vi "Add Attribute To Tree.vi"(6 "Display Name":string="Root::AcquisitionControl::AcquisitionStart", 8 "Error In":errorcluster, 9 "Active Item:Symbol Index":i32, 10 "Attribute Name":string="Root::AcquisitionControl::AcquisitionStart", 11 "Attribute Table In":refnum<vi>) -> (0 "Error Out":errorcluster, 3 "Attribute Table Out":refnum<vi>)   [LabVIEW 2018, in "TraceTreeEditor.lvlib"]
uses:
  TraceTreeEditor.lvlib
panel:
  out "Navigate Tree:Get Parent":string
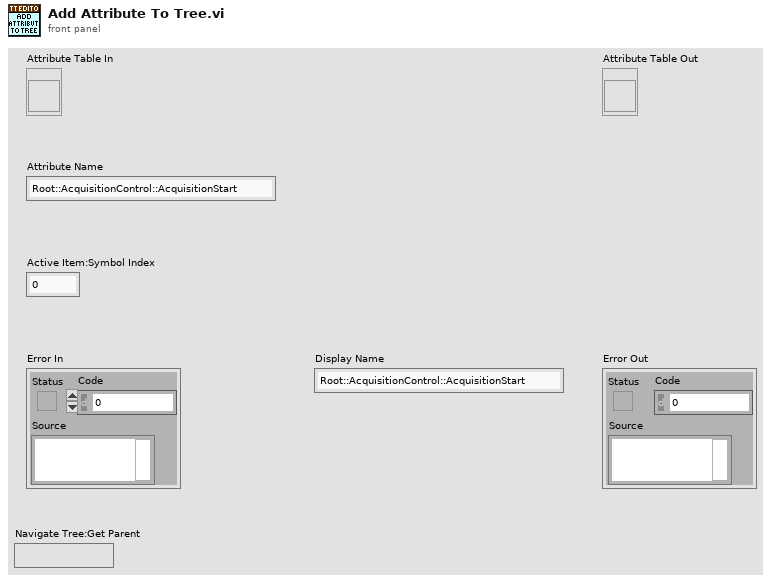
[diagram p1: front panel]
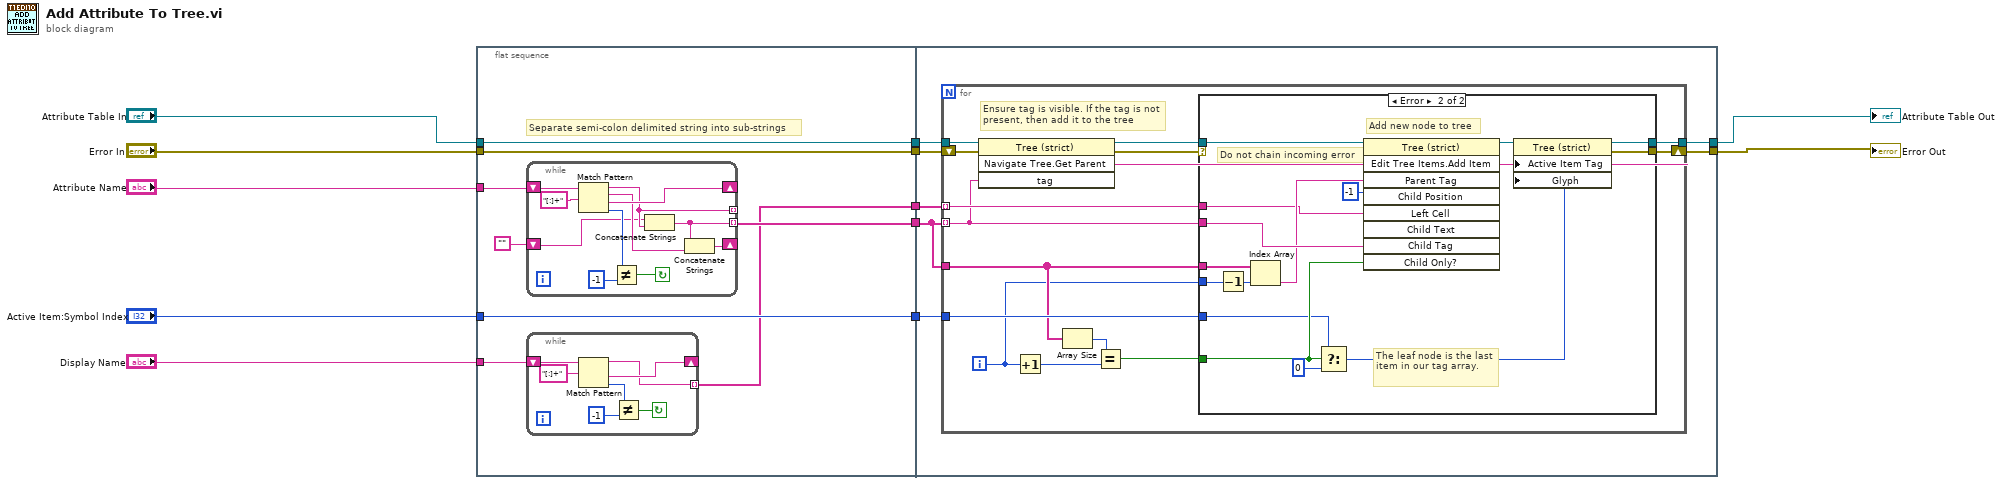
[diagram p0: block diagram]
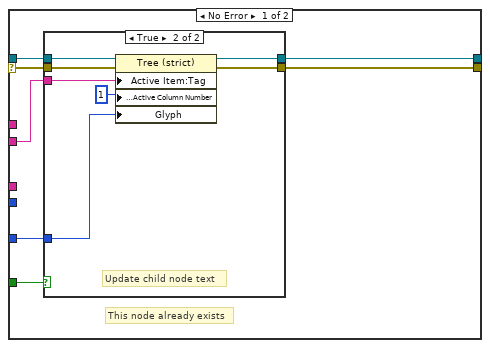
[diagram p2: hidden frame]
diagram:
  n1 = flat-sequence {
    tunnel: "Attribute Name" -> [w18]
    tunnel: [w17] -> w8
    tunnel: [w13] -> w7
    tunnel: "Attribute Table In" -> [w16]
    tunnel: [w16] -> w6
    tunnel: "Error In" -> [w20]
    tunnel: [w20] -> w12
    tunnel: "Active Item:Symbol Index" -> [w15]
    tunnel: [w15] -> w3
    tunnel: "Display Name" -> [w14]
    tunnel: w8 -> [w41]
    tunnel: w7 -> [w42]
    tunnel: w6 -> [w43]
    tunnel: w12 -> [w45]
    tunnel: [w44] -> w11
    tunnel: [w40] -> w5
    tunnel: w3 -> [w39]
    frame #0 {
      # "Separate semi-colon delimited string into sub-strings"
      n2 = while {
        shift-right: [w35] -> _
        shift-left: w18 -> [w34]
        tunnel: [w29] -> _ mode=indexing
        shift-right: [w31] -> _
        shift-left: "" -> [w28]
        tunnel: [w32] -> w17 mode=indexing
        stop <- w37 continue-if-true
        n3 = Match Pattern(string=w34, regular expression="[:]+") -> (before substring=w29:string, match substring=w30:string, after substring=w35:string, offset past match=w33:i32)  [unwired: 1 out]
        n4 = Not Equal?(x=w33, y=-1) -> (x != y?=w37:bool)
        n5 = Concatenate Strings(w28, w29) -> (w32:string)
        n6 = Concatenate Strings(w32, w30) -> (w31:string)
      }
      n7 = while {
        shift-right: [w24] -> _
        shift-left: w14 -> [w23]
        tunnel: [w21] -> w13 mode=indexing
        stop <- w26 continue-if-true
        n8 = Match Pattern(string=w23, regular expression="[:]+") -> (before substring=w21:string, after substring=w24:string, offset past match=w22:i32)  [unwired: 2 out]
        n9 = Not Equal?(x=w22, y=-1) -> (x != y?=w26:bool)
      }
    }
    frame #1 {
      n10 = for {
        tunnel: w41 -> [w53] mode=indexing
        tunnel: w43 -> [w57]
        tunnel: [w55] -> w40
        tunnel: w42 -> [w54] mode=indexing
        shift-right: [w58] -> w44
        shift-left: w45 -> [w59]
        tunnel: w41 -> [w48]
        tunnel: w39 -> [w52]
        i -> [w46]
        # "Ensure tag is visible. If the tag is not present, then add it to the tree"
        n11 = invoke class="Tree (strict)" method="Navigate Tree.Get Parent"(reference=w57, error in=w59, "tag"=w53) -> (reference out=w56:refnum<vi>, error out=w60:errorcluster, "Navigate Tree:Get Parent"=→"Navigate Tree:Get Parent":string)  [unwired: 1 in, 1 out]
        n12 = Increment(x=w46) -> (x+1=w50:i32)
        n13 = Array Size(array=w48) -> (size(s)=w51:i32)
        n14 = Equal?(x=w51, y=w50) -> (x = y?=w49:bool)
        n15 = case shown="Error" w60 {
          selector: w60 -> [w67 _]
          tunnel: w56 -> [w65 w91]
          tunnel: [w64 w80] -> w55
          tunnel: [w66 w92] -> w58
          tunnel: w54 -> [_ w81]
          tunnel: w53 -> [w62 w89]
          tunnel: w48 -> [_ w83]
          tunnel: w52 -> [w61 w77]
          tunnel: w46 -> [_ w85]
          tunnel: w49 -> [w63 w82]
          frame No Error {
            # "This node already exists"
            n16 = case shown="True" w63 {
              tunnel: w65 -> [w68 w74]
              tunnel: [w68 w73] -> w64
              tunnel: w67 -> [w69 w76]
              tunnel: [w69 w75] -> w66
              tunnel: w62 -> [_ w72]
              tunnel: w61 -> [_ w70]
              frame False {
              }
              frame True {
                # "Update child node text"
                n17 = property class="Tree (strict)"(reference=w74, error in=w76, "Active Item:Tag"=w72, "Active Cell:Active Column Number"=1 ("Active Cell Properties:Active Column Number"), "Glyph"=w70) -> (reference out=w73:refnum<vi>, error out=w75:errorcluster)
              }
            }
          }
          frame Error {
            # "Add new node to tree"
            # "The leaf node is the last item in our tag array."
            # "Do not chain incoming error"
            n18 = Decrement(x=w85) -> (x-1=w86:i32)
            n19 = Index Array(array=w83, index=w86) -> (element=w84:string)
            n20 = Select(t=w77, s=w82, f=0) -> (s? t:f=w78:i32)
            n21 = invoke class="Tree (strict)" method="Edit Tree Items.Add Item"(reference=w91, "Parent Tag"=w84, "Child Position"=-1, "Left Cell"=w81, "Child Tag"=w89, "Child Only?"=w82) -> (reference out=w90:refnum<vi>, "Edit Tree Items:Add Item"=w79:string)  [unwired: 3 in, 7 out]
            n22 = property class="Tree (strict)"(reference=w90, "Active Item Tag"=w79, "Glyph"=w78) -> (reference out=w80:refnum<vi>, error out=w92:errorcluster)  [unwired: 1 in]
          }
        }
      }
    }
  }
  "Error Out" <- w11
  "Attribute Table Out" <- w5
